vi "DSF.Engine.Interface.Builder.Read.vi"   [LabVIEW 2016, in "DSF.Engine.lvlib" / "DSF.Engine.Interface.Builder.lvclass"]
uses:
  DSF.Engine.Interface.Builder.lvclass
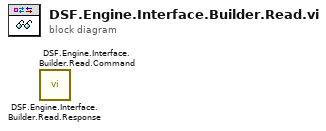
[diagram p0: block diagram]
diagram:
  n1 = call "DSF.Engine.Interface.Builder.Read.Response.vi"() -> ()  [unwired: 7 in, 5 out]
  n2 = call "DSF.Engine.Interface.Builder.Read.Command.vi"() -> ()  [unwired: 7 in, 5 out]
